vi "HandShaking.vi"(6 "Elapsed Time":u32, 8 "error in":errorcluster, 9 "Sequence Context":refnum<k7>, 10 "Stop":refnum<user-event>, 11 "TestExec in":refnum<class "TestExec.lvclass">) -> (0 "error out":errorcluster, 3 "TestExec out":refnum<class "TestExec.lvclass">)   [LabVIEW 2019, in "OPC UA.lvlib" / "TestExec.lvclass"]
uses:
  TestExec.lvclass
  C:/Workspace/BSM OOP/Sequence/CodeModules/OPC UA Client/OPC UA/OPC UA.lvclass
  OPC UA/OPC UA.lvclass/OPC UA.ctl
  TestExec.lvclass/TestExec.ctl
  40e5e5ce-79b7-40ff-98c1-3a323906afd5.vi
  <vilib>/addons/TestStand/_TSUtility.llb/TestStand - Get Property Value (Number {Signed 32-bit Integer}).vi
  OPC UA/OPC UA.lvclass
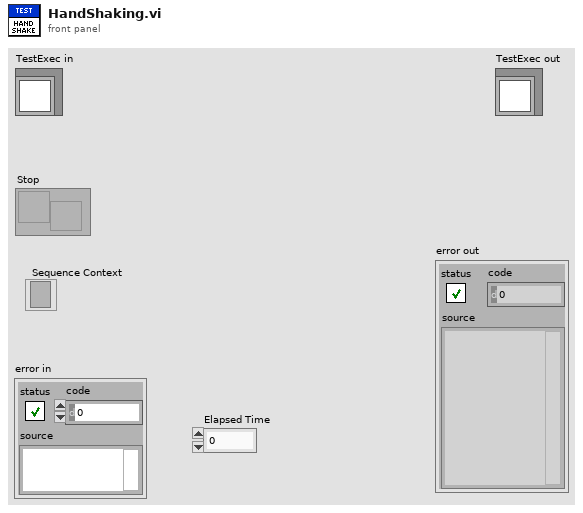
[diagram p1: front panel]
types:
  T1 = typedef "OPC UA.lvlib/OPC UA.lvclass/Tester Tx Dataset.ctl" = cluster{"Fault":bool, "StepNo":u32, "Ready":bool, "HighVoltage":bool, "TestRunning":bool, "ResultsReady":bool, "Results":u32, "ElapsedTime":u32, "Online":bool, "TimeCompleted":i32[], "Timeout":bool, "Heartbeat":bool}
  T2 = typedef "OPC UA.lvlib/OPC UA.lvclass/Tester Rx Dataset.ctl" = cluster{"Start":bool, "NestStatus":bool, "PalletID":u32, "BarcodeData":string, "StepEcho":u32, "Cylinder_1":bool, "Cylinder_2":bool, "Cylinder_3":bool, "Cylinder_4":bool, "Cylinder_5":bool, "ResultsAck":bool, "Reset":bool, "Stop":bool, "FaultCode":u32}
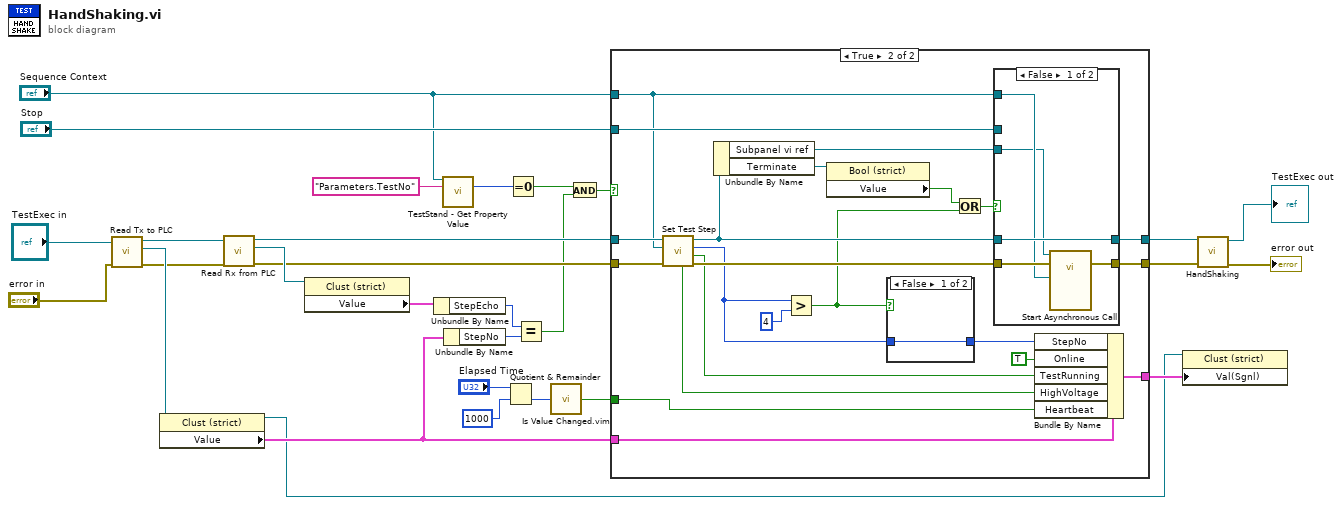
[diagram p0: block diagram]
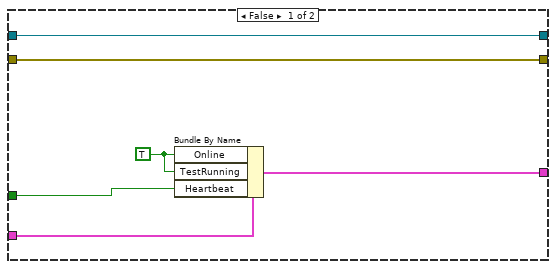
[diagram p2: hidden frame]
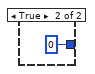
[diagram p3: hidden frame]
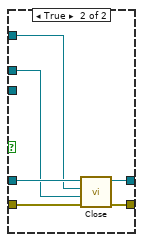
[diagram p4: hidden frame]
diagram:
  n1 = call "Read Tx to PLC.vi"("error in (no error)"="error in", "OPC UA in"="TestExec in") -> ("error out"=w9:errorcluster, "Tx to PLC"=w23:refnum<vi>, "OPC UA out"=w12:refnum<class "TestExec.lvclass">)  [unwired: 7 in]
  n2 = property on="Property Node" class="Clust (strict)"(reference=w23) -> (reference out=w1:refnum<vi>, "Value"=w2:T1)  [unwired: 1 in, 1 out]
  n3 = call "Read Rx from PLC.vi"("error in (no error)"=w9, "OPC UA in"=w12) -> ("error out"=w8:errorcluster, "Rx from PLC"=w22:refnum<vi>, "OPC UA out"=w11:refnum<class "TestExec.lvclass">)  [unwired: 7 in]
  n4 = property on="Property Node" class="Clust (strict)"(reference=w22) -> ("Value"=w27:T2)  [unwired: 1 in, 2 out]
  n5 = Unbundle By Name(w27) -> ("StepEcho"=w7:u32)
  n6 = call-poly <vilib>:"TestStand - Get Property Value.vi"("Sequence Context In"="Sequence Context", "Lookup String"="Parameters.TestNo") -> ("Value"=w24:i32)  [unwired: 11 in, 2 out]
  n7 = Unbundle By Name(w2) -> ("StepNo"=w6:u32)
  n8 = Quotient & Remainder(x="Elapsed Time", y=u32 1000) -> (floor(x/y)=w18:u32)  [unwired: 1 out]
  n9 = Equal To 0?(x=w24) -> (x = 0?=w4:bool)
  n10 = Equal?(x=w7, y=w6) -> (x = y?=w3:bool)
  n11 = call "Is Value Changed.vim"("value"=w18) -> ("changed or first call?"=w16:bool)
  n12 = And(x=w4, y=w3) -> (x .and. y?=w25:bool)
  n13 = case shown="True" w25 {
    tunnel: w2 -> [w34 w44]
    tunnel: "Sequence Context" -> [_ w39]
    tunnel: "Stop" -> [_ w53]
    tunnel: w11 -> [w35 w56]
    tunnel: [w35 w54] -> w20
    tunnel: w16 -> [w31 w43]
    tunnel: [w33 w40] -> w15
    tunnel: [w30 w51] -> w14
    tunnel: w8 -> [w30 w50]
    frame False {
      w32 = TRUE ("Online")
      n14 = Bundle By Name(cluster=w34, "Online"=w32, "TestRunning"=w32, "Heartbeat"=w31) -> (w33:T1)
    }
    frame True {
      n15 = call "Set Test Step .vi"("error in (no error)"=w50, "Sequence Context In"=w39, "TestExec.lvclass"=w56) -> ("error out"=w52:errorcluster, "Test Running"=w42:bool, "Next Step"=w37:i32, "TestExec.lvclass"=w49:refnum<class "TestExec.lvclass">, "HV"=w41:bool)  [unwired: 4 in]
      n16 = Unbundle By Name(w49) -> ("Subpanel vi ref"=w48:refnum<vi>, "Terminate"=w47:refnum<vi>)
      n17 = Greater?(x=w37, y=4) -> (0:w38:bool)
      n18 = property class="Bool (strict)"(reference=w47) -> ("Value"=w46:bool)  [unwired: 1 in, 2 out]
      n19 = case shown="False" w38 {
        tunnel: w37 -> [w58 _]
        tunnel: [w58 0 ("Next Step")] -> w36
        frame False {
        }
        frame True {
        }
      }
      n20 = Or(x=w46, y=w38) -> (x .or. y?=w45:bool)
      n21 = case shown="False" w45 {
        tunnel: w49 -> [w64 w70]
        tunnel: [w64 w69] -> w54
        tunnel: w53 -> [_ w68]
        tunnel: w39 -> [w61 w67]
        tunnel: w52 -> [w63 w66]
        tunnel: [w62 w65] -> w51
        tunnel: w48 -> [w60 _]
        frame False {
          n22 = call-by-ref "Start Asynchronous Call"(reference=w60, error in=w63, "Sequence Context"=w61) -> (error out=w62:errorcluster)  [unwired: 10 in, 2 out]
        }
        frame True {
          n23 = call-dynamic "Close.vi"("error in (no error)"=w66, "Stop Event"=w68, "Sequence Context"=w67, "TestExec in"=w70) -> ("error out"=w65:errorcluster, "TestExec out"=w69:refnum<class "TestExec.lvclass">)  [unwired: 6 in]
        }
      }
      n24 = Bundle By Name(cluster=w44, "StepNo"=w36, "Online"=TRUE, "TestRunning"=w42, "HighVoltage"=w41, "Heartbeat"=w43) -> (w40:T1)
    }
  }
  n25 = property on="Property Node" class="Clust (strict)"(reference=w1, "Val(Sgnl)"=w15) -> ()  [unwired: 1 in, 2 out]
  n26 = call-parent "HandShaking.vi"("error in (no error)"=w14, "OPC UA in"=w20) -> ("error out"=→"error out":errorcluster, "OPC UA out"=→"TestExec out":refnum<class "TestExec.lvclass">)  [unwired: 8 in]
